vi "introduction.vi"() -> ()   [LabVIEW 2014]
uses:
  builds/LVTables/SQLite Packed/SQLite3LV.lvlibp/Cursor Class/property binding/bind text.vi
  builds/LVTables/SQLite Packed/SQLite3LV.lvlibp/Cursor Class/property binding/column Text.vi
  builds/LVTables/SQLite Packed/SQLite3LV.lvlibp/SQLite3 Class/sqlite3.lvclass
  builds/LVTables/SQLite Packed/SQLite3LV.lvlibp/Cursor Class/cursor.lvclass
panel:
  out "error out":errorcluster
  out "Last Names":string[](array[string])
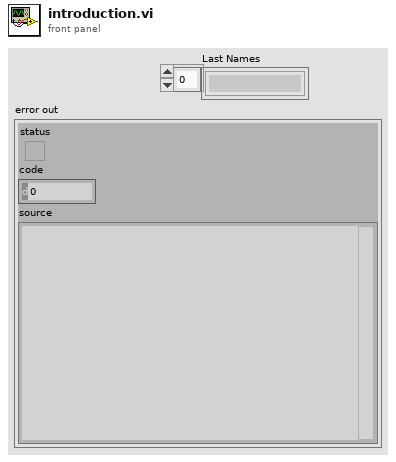
[diagram p1: front panel]
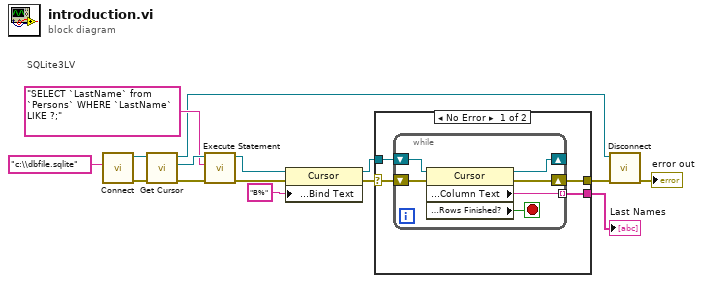
[diagram p0: block diagram]
diagram:
  # "SQLite3LV"
  n1 = call "Connect.vi"("path"="c:\\dbfile.sqlite") -> ("error out"=w10:errorcluster, "SQLite3LV Connection out"=w15:refnum<class "sqlite3.lvclass">)  [unwired: 9 in]
  n2 = call "Get Cursor.vi"("error in (no error)"=w10, "SQLite3LV Connection in"=w15) -> ("error out"=w9:errorcluster, "SQLite3LV Cursor"=w14:refnum<class "cursor.lvclass">, "SQLite3LV Connection out"=w7:refnum<class "sqlite3.lvclass">)  [unwired: 7 in]
  n3 = call "Execute Statement.vi"("error in (no error)"=w9, "SQL statement"="SELECT `LastName` from `Persons` WHERE `LastName` LIKE ?;", "SQLite3LV Cursor in"=w14) -> ("error out"=w4:errorcluster, "SQLite3LV Cursor out"=w12:refnum<class "cursor.lvclass">)  [unwired: 7 in]
  n4 = property class="Cursor"(reference=w12, error in=w4, "property binding:Bind Text"="B%" ("Bind Text")) -> (reference out=w6:refnum<class "cursor.lvclass">, error out=w3:errorcluster)
  n5 = case shown="No Error" w3 {
    selector: w3 -> [w16 w26]
    tunnel: [w19 _] -> w11
    tunnel: [w18 w26] -> w8
    tunnel: w6 -> [w17 _]
    frame No Error {
      n6 = while {
        shift-right: [w22] -> _
        shift-left: w17 -> [w25]
        shift-right: [w23] -> w18
        shift-left: w16 -> [w24]
        tunnel: [w20] -> w19 mode=indexing
        stop <- w21 stop-if-true
        n7 = property class="Cursor"(reference=w25, error in=w24) -> (reference out=w22:refnum<class "cursor.lvclass">, error out=w23:errorcluster, "property binding:Column Text"=w20:string, "property binding:Rows Finished?"=w21:bool)
      }
    }
    frame Error {
    }
  }
  "Last Names" <- w11
  n8 = call "Disconnect.vi"("error in (no error)"=w8, "SQLite3LV Connection in"=w7) -> ("error out"=→"error out":errorcluster)  [unwired: 9 in]
